vi "Msg.vi"(7 "jettl in":refnum<class "jettl.lvclass">, 11 "Setup Msg Strategy in":refnum<class "Setup Msg Strategy.lvclass">) -> (5 "jettl out":refnum<class "jettl.lvclass">)   [LabVIEW 2021, in "jettl Msg Setup.lvlib" / "Setup Msg Strategy.lvclass"]
uses:
  Setup Msg Strategy.lvclass
  jettl/jettl/jettl.lvclass
  Setup/Setup.lvclass
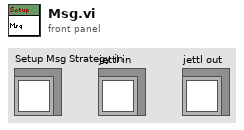
[diagram p1: front panel]
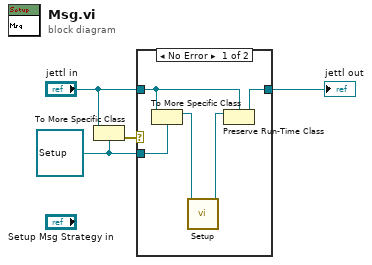
[diagram p0: block diagram]
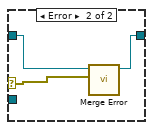
[diagram p2: hidden frame]
diagram:
  w2 = refnum<class "Setup.lvclass"> refnum ("Setup.lvlib:Setup.lvclass")
  n1 = To More Specific Class(target class=w2, reference="jettl in") -> (error out=w4:errorcluster)  [unwired: 1 in, 1 out]
  n2 = case shown="No Error" w4 {
    selector: w4 -> [_ w11]
    tunnel: [w7 w10] -> w1
    tunnel: "jettl in" -> [w8 w12]
    tunnel: w2 -> [w9 _]
    frame No Error {
      n3 = To More Specific Class(target class=w9, reference=w8) -> (specific class reference=w6:refnum<class "Setup.lvclass">)  [unwired: 1 in, 1 out]
      n4 = call-dynamic "Setup.vi"("Setup in"=w6) -> ("Setup out"=w5:refnum<class "Setup.lvclass">)  [unwired: 10 in]
      n5 = Preserve Run-Time Class(object in=w5, 2:w8) -> (object out=w7:refnum<class "jettl.lvclass">)  [unwired: 1 in, 1 out]
    }
    frame Error {
      n6 = call-dynamic "Merge Error.vi"("Error"=w11, "Merge Error in"=w12) -> ("Merge Error out"=w10:refnum<class "jettl.lvclass">)  [unwired: 9 in]
    }
  }
  "jettl out" <- w1
